vi "Streaming Message Loop.vi"(8 "error in (no error)":errorcluster, 9 "notifier out":refnum<notifier>, 10 "queue out":refnum<queue>, 11 "Message Queues":T1) -> (0 "error out":errorcluster)   [LabVIEW 2024]
doc: "The message loop subVI to handle messages pertaining to logging data."
uses:
  support/Message Queue/All Message Queues.ctl
  support/Message Queue/Message Cluster.ctl
  controls/DAQ_msgHandler StreamTypeDef.ctl
  CTRsample/Control/streamIO_states.ctl
  <vilib>/Utility/error.llb/Error Cluster From Error Code.vi
  <vilib>/ErrorRing/Error Ring.xnode
  support/Message Queue/DAQ_msgHandler Message Queue.lvlib
  Logging/DAQ_msgHandler Logging.lvlib
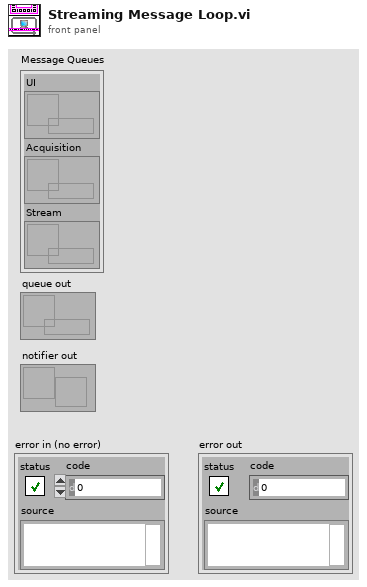
[diagram p1: front panel]
types:
  T1 = typedef "DAQ_msgHandler Message Queue.lvlib/All Message Queues.ctl" = cluster{"UI":refnum<queue>, "Acquisition":refnum<queue>, "Stream":refnum<queue>}
  T2 = typedef "streamIO_states.ctl" = enum16{"Fault", "Initialize", "Stream", "Close"}
  T3 = typedef "DAQ_msgHandler StreamTypeDef.ctl" = cluster{"stream state":T2, "CTR Node":string, "DAQ Node ID":i32, "Writer Endpoint":refnum<k21>, "Reader Endpoint":refnum<k21>, "Buffer":i32, "Managment Timeout":i32, "Stream Timeout":i32, "DAQ IP Addr":string, "CTR IP Addr":string, "Timeout Counter":i32}
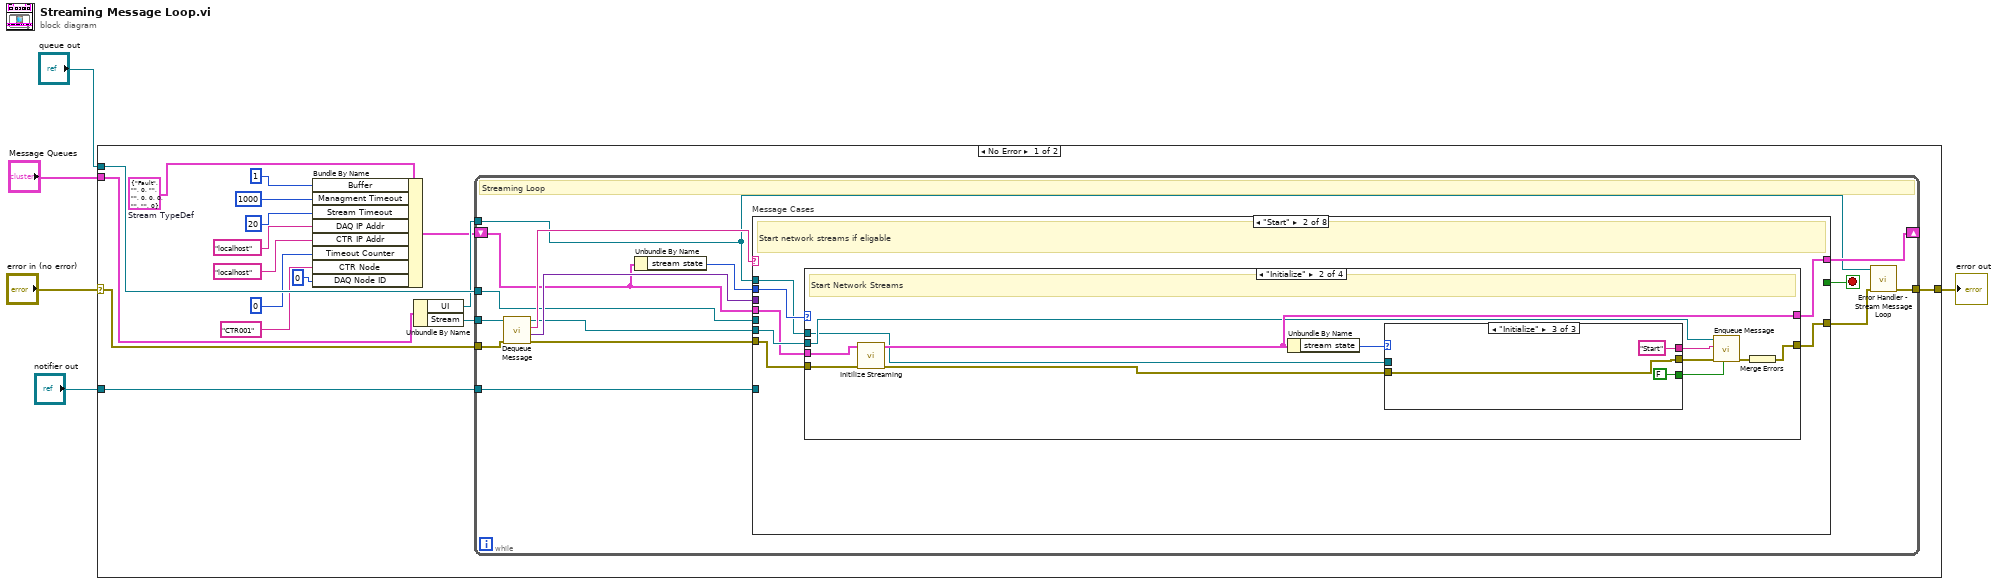
[diagram p0: block diagram]
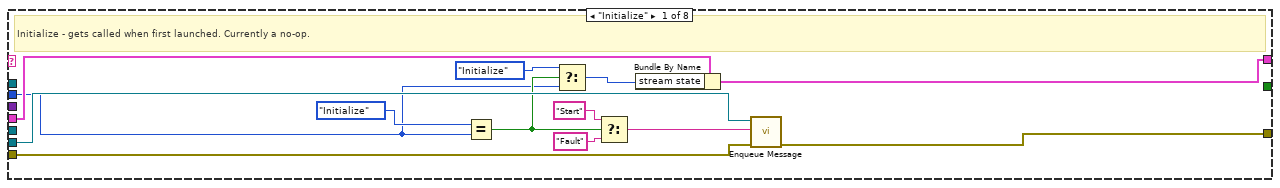
[diagram p2: hidden frame]
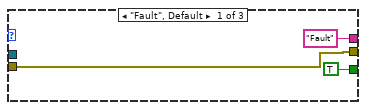
[diagram p4: hidden frame]
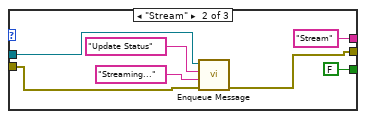
[diagram p5: hidden frame]
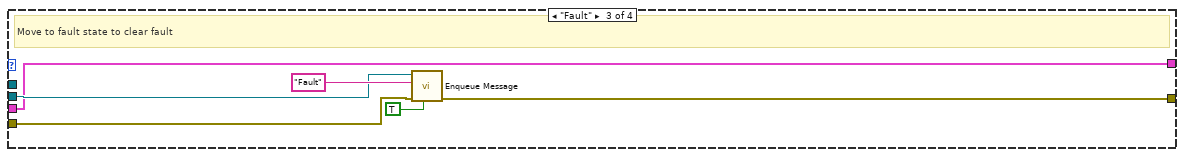
[diagram p6: hidden frame]
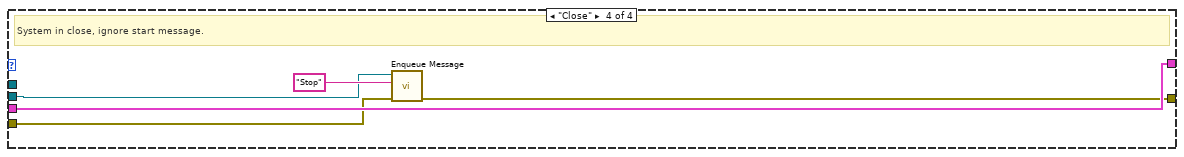
[diagram p7: hidden frame]
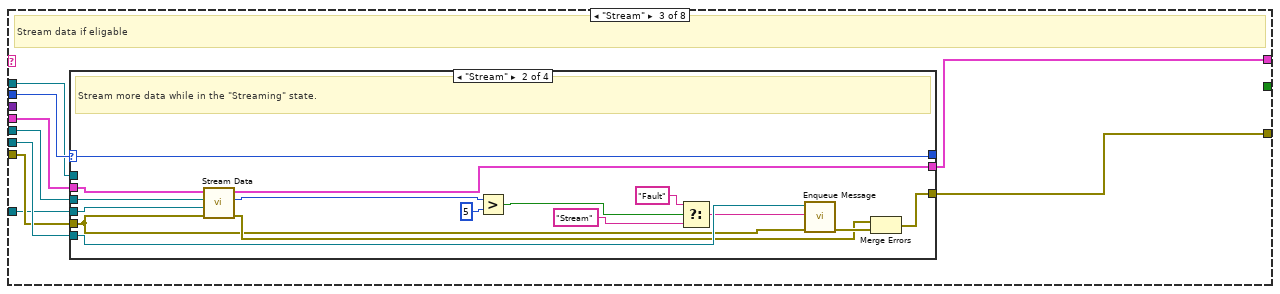
[diagram p8: hidden frame]
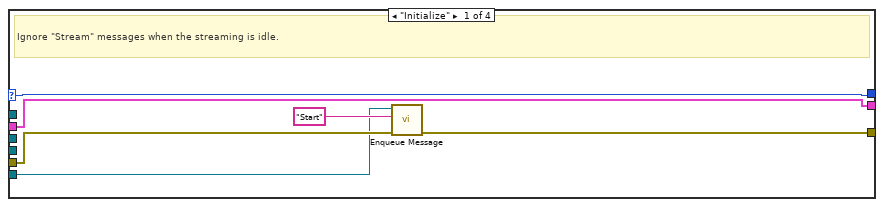
[diagram p9: hidden frame]
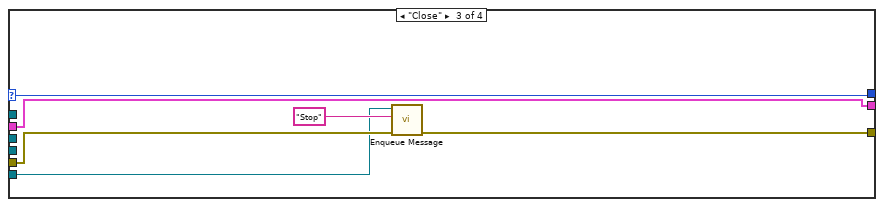
[diagram p10: hidden frame]
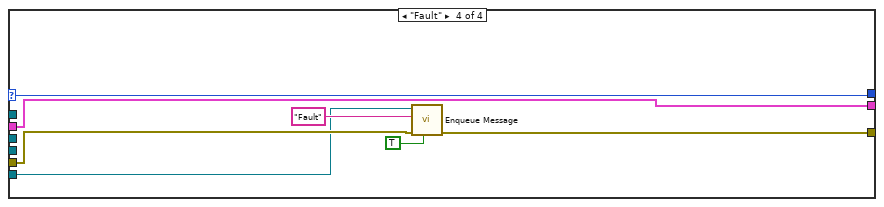
[diagram p11: hidden frame]
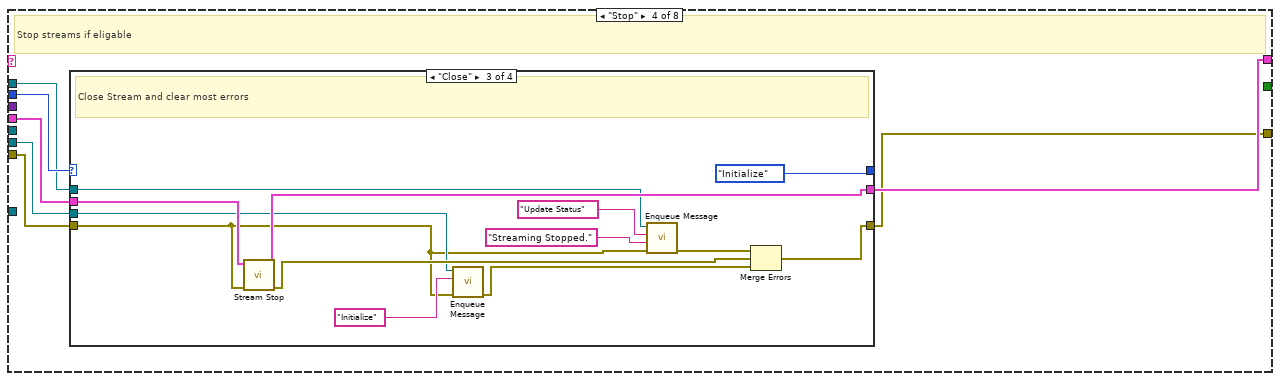
[diagram p12: hidden frame]
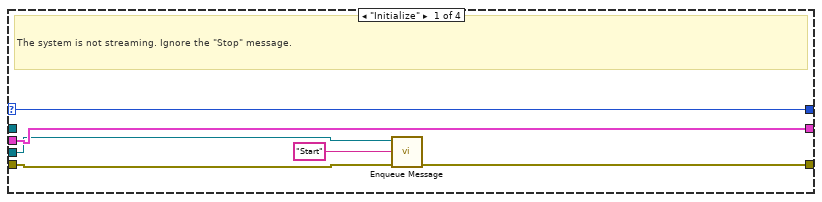
[diagram p13: hidden frame]
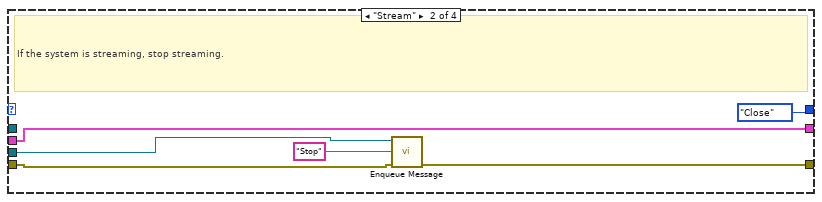
[diagram p14: hidden frame]
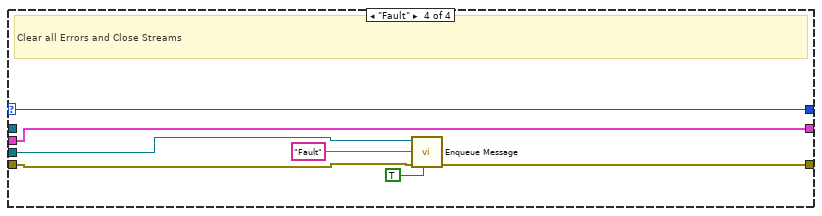
[diagram p15: hidden frame]
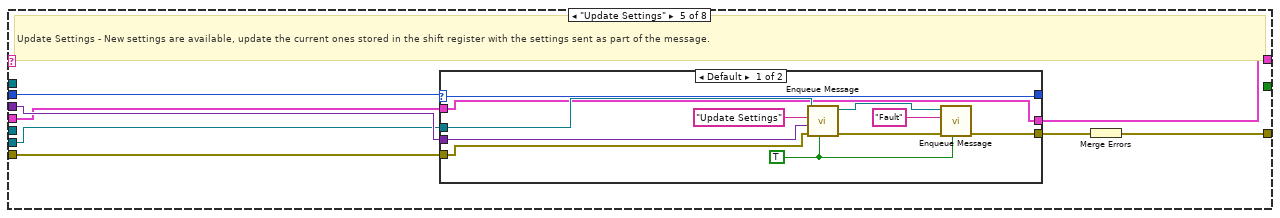
[diagram p16: hidden frame]
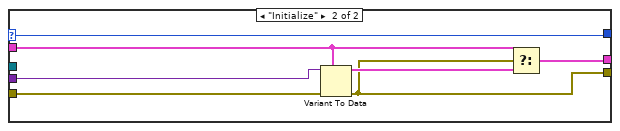
[diagram p17: hidden frame]
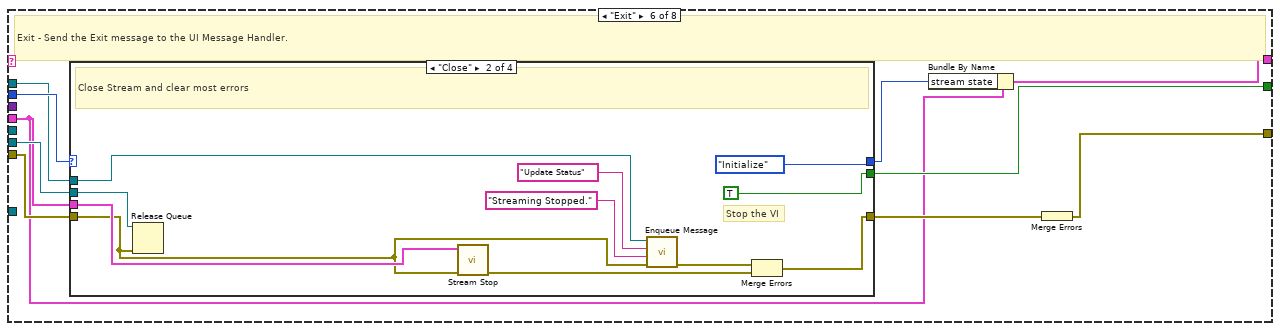
[diagram p18: hidden frame]
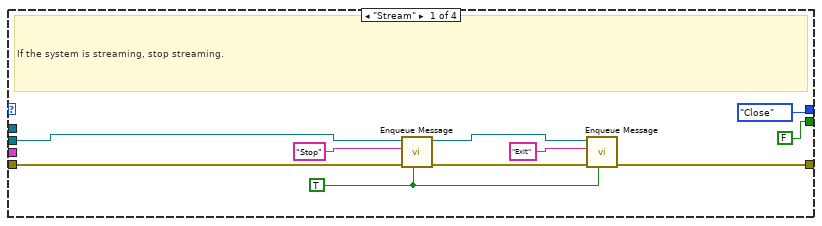
[diagram p19: hidden frame]
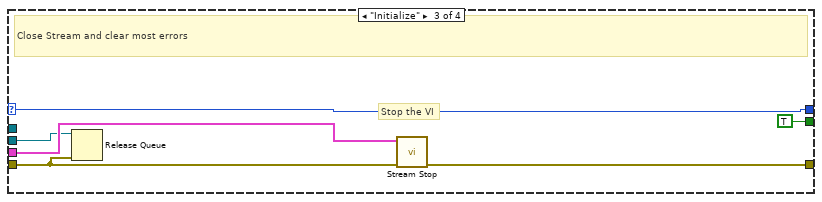
[diagram p20: hidden frame]
diagram:
  n1 = case shown="No Error" "error in (no error)" {
    selector: "error in (no error)" -> [w19 w286]
    tunnel: "Message Queues" -> [w22 _]
    tunnel: [w20 w286] -> w4
    tunnel: "queue out" -> [w18 _]
    tunnel: "notifier out" -> [w16 _]
    frame No Error {
      w15 = T3 {"stream state"=enum."Fault", "CTR Node"="", "DAQ Node ID"=0, "Writer Endpoint"="", "Reader Endpoint"="", "Buffer"=0, "Managment Timeout"=0, "Stream Timeout"=0, "DAQ IP Addr"="", "CTR IP Addr"="", "Timeout Counter"=0}  # Stream TypeDef
      n2 = Bundle By Name(cluster=w15, "Buffer"=1, "Managment Timeout"=1000, "Stream Timeout"=20, "DAQ IP Addr"="localhost", "CTR IP Addr"="localhost", "Timeout Counter"=0, "CTR Node"="CTR001", "DAQ Node ID"=0) -> (w14:T3)
      n3 = Unbundle By Name(w22) -> ("UI"=w17:refnum<queue>, "Stream"=w21:refnum<queue>)
      n4 = while {
        tunnel: w21 -> [w31]
        shift-right: [w25] -> _
        shift-left: w14 -> [w27]
        tunnel: w17 -> [w24]
        tunnel: w18 -> [w30]
        tunnel: w19 -> [w36]
        tunnel: [w29] -> w20
        tunnel: w16 -> [w28]
        stop <- w37 stop-if-true
        # "Streaming Loop"
        n5 = call "Dequeue Message.vi"("error in (no error)"=w36, "Message Queue"=w31) -> ("error out"=w35:errorcluster, "Message Data"=w33:variant, "Message"=w34:string, "dup Message Queue"=w32:refnum<queue>)  [unwired: 6 in]
        n6 = Unbundle By Name(w27) -> ("stream state"=w26:T2)
        n7 = case "Message Cases" shown="\"Start\"" w34 {
          selector: w34 -> [_ _ _ _ _ _ _ w277]
          tunnel: w32 -> [w48 w56 w103 w143 w180 w211 w262 w272]
          tunnel: w35 -> [w50 w55 w101 w145 w182 w212 w267 w276]
          tunnel: [w49 w57 w104 w141 w186 w214 w270 w275] -> w23
          tunnel: w27 -> [w47 w54 w100 w146 w184 w208 w268 w278]
          tunnel: [w46 w53 w97 w142 w183 w207 w265 w278] -> w25
          tunnel: [_ _ _ _ _ w210 _ _] -> w37
          tunnel: w33 -> [_ _ _ _ w185 _ _ _]
          tunnel: w30 -> [_ _ w102 _ _ _ _ _]
          tunnel: w26 -> [w39 w52 w99 w144 w181 w213 _ _]
          tunnel: w28 -> [_ _ w98 _ _ _ _ _]
          tunnel: w24 -> [_ w51 w96 w140 _ w205 w255 _]
          frame "Initialize" {
            # "Initialize - gets called when first launched. Currently a no-op."
            n8 = Equal?(x=streamIO_states."Initialize", y=w39) -> (x = y?=w40:bool)
            n9 = Select(t=streamIO_states."Initialize" ("stream state"), s=w40, f=w39) -> (s? t:f=w38:T2)
            n10 = Select(t="Start" ("Message"), s=w40, f="Fault") -> (s? t:f=w42:string)
            n11 = Bundle By Name(cluster=w47, "stream state"=w38) -> (w46:T3)
            n12 = call-poly "Enqueue Message.vi"("error in (no error)"=w50, "Message"=w42, "Message Queue"=w48) -> ("error out"=w49:errorcluster)  [unwired: 7 in, 1 out]
          }
          frame "Start" {
            # "Start network streams if eligable"
            n13 = case shown="\"Initialize\"" w52 {
              tunnel: [w58 w69 w87 w91] -> w57
              tunnel: w56 -> [_ w64 w89 w92]
              tunnel: w55 -> [w58 w68 w88 w93]
              tunnel: w54 -> [w59 w67 w85 w95]
              tunnel: [w59 w66 w85 w95] -> w53
              tunnel: w51 -> [_ w60 _ _]
              frame "Stream" {
                # "The system is already Streaming. Ignore the \"Start\" message."
              }
              frame "Initialize" {
                # "Start Network Streams"
                n14 = call "Initilize Streaming.vi"("error in (no error)"=w68, "DAQ_msgHandler StreamTypeDef"=w67) -> ("error out"=w62:errorcluster, "DAQ_msgHandler StreamTypeDef 2"=w66:T3)  [unwired: 8 in]
                n15 = Unbundle By Name(w66) -> ("stream state"=w65:T2)
                n16 = case shown="\"Initialize\"" w65 {
                  tunnel: ["Fault" ("Message") "Stream" ("Message") "Start" ("Message")] -> w71
                  tunnel: [TRUE ("Priority Message? (F)") FALSE ("Priority Message? (F)") FALSE ("Priority Message? (F)")] -> w63
                  tunnel: w62 -> [w72 w77 w82]
                  tunnel: [w72 w76 w82] -> w61
                  tunnel: w60 -> [_ w75 _]
                  frame "Fault", Default {
                  }
                  frame "Stream" {
                    n17 = call-poly "Enqueue Message.vi"("error in (no error)"=w77, "Message Data"="Streaming..." ("Acquiring and Logging..."), "Message"="Update Status", "Message Queue"=w75) -> ("error out"=w76:errorcluster)  [unwired: 6 in, 1 out]
                  }
                  frame "Initialize" {
                  }
                }
                n18 = call-poly "Enqueue Message.vi"("Priority Message? (F)"=w63, "error in (no error)"=w61, "Message"=w71, "Message Queue"=w64) -> ("error out"=w70:errorcluster)  [unwired: 6 in, 1 out]
                n19 = Merge Errors(w70) -> (w69:errorcluster)
              }
              frame "Fault" {
                # "Move to fault state to clear fault"
                n20 = call-poly "Enqueue Message.vi"("Priority Message? (F)"=TRUE, "error in (no error)"=w88, "Message"="Fault", "Message Queue"=w89) -> ("error out"=w87:errorcluster)  [unwired: 6 in, 1 out]
              }
              frame "Close" {
                # "System in close, ignore start message."
                n21 = call-poly "Enqueue Message.vi"("error in (no error)"=w93, "Message"="Stop", "Message Queue"=w92) -> ("error out"=w91:errorcluster)  [unwired: 7 in, 1 out]
              }
            }
          }
          frame "Stream" {
            # "Stream data if eligable"
            n22 = case shown="\"Stream\"" w99 {
              selector: w99 -> [w110 w121 w131 w138]
              tunnel: [w105 w126 w127 w133] -> w104
              tunnel: w103 -> [w106 w124 w128 w134]
              tunnel: w102 -> [_ w123 _ _]
              tunnel: w101 -> [w107 w111 w129 w135]
              tunnel: w100 -> [w109 w120 w132 w139]
              tunnel: [w110 w121 w131 w138] -> _
              tunnel: w98 -> [_ w119 _ _]
              tunnel: [w109 w118 w132 w139] -> w97
              tunnel: w96 -> [_ _ _ _]
              frame "Initialize" {
                # "Ignore \"Stream\" messages when the streaming is idle."
                n23 = call-poly "Enqueue Message.vi"("error in (no error)"=w107, "Message"="Start", "Message Queue"=w106) -> ("error out"=w105:errorcluster)  [unwired: 7 in, 1 out]
              }
              frame "Stream" {
                # "Stream more data while in the \"Streaming\" state."
                n24 = call "Stream Data.vi"("error in (no error)"=w111, "notifier out"=w119, "queue out"=w123, "DAQ_msgHandler StreamTypeDef"=w120) -> ("error out"=w122:errorcluster, "Timout Counter"=w112:i32, "DAQ_msgHandler StreamTypeDef 2"=w118:T3)  [unwired: 5 in]
                n25 = Greater?(x=w112, y=5 ("x")) -> (0:w116:bool)
                n26 = Select(t="Fault", s=w116, f="Stream" ("Message")) -> (s? t:f=w114:string)
                n27 = call-poly "Enqueue Message.vi"("error in (no error)"=w111, "Message"=w114, "Message Queue"=w124) -> ("error out"=w125:errorcluster)  [unwired: 7 in, 1 out]
                n28 = Merge Errors(w122, w125) -> (w126:errorcluster)
              }
              frame "Close" {
                n29 = call-poly "Enqueue Message.vi"("error in (no error)"=w129, "Message"="Stop", "Message Queue"=w128) -> ("error out"=w127:errorcluster)  [unwired: 7 in, 1 out]
              }
              frame "Fault" {
                n30 = call-poly "Enqueue Message.vi"("Priority Message? (F)"=TRUE, "error in (no error)"=w135, "Message"="Fault", "Message Queue"=w134) -> ("error out"=w133:errorcluster)  [unwired: 6 in, 1 out]
              }
            }
          }
          frame "Stop" {
            # "Stop streams if eligable"
            n31 = case shown="\"Close\"" w144 {
              selector: w144 -> [w152 _ _ w174]
              tunnel: [w148 w155 w168 w173] -> w141
              tunnel: w146 -> [w151 w153 w170 w172]
              tunnel: w145 -> [w149 w156 w161 w176]
              tunnel: [w152 streamIO_states."Close" ("stream state") streamIO_states."Initialize" ("stream state") w174] -> _
              tunnel: w143 -> [w147 w154 w165 w175]
              tunnel: [w151 w153 w169 w172] -> w142
              tunnel: w140 -> [_ _ w160 _]
              frame "Initialize" {
                # "The system is not streaming. Ignore the \"Stop\" message."
                n32 = call-poly "Enqueue Message.vi"("error in (no error)"=w149, "Message"="Start", "Message Queue"=w147) -> ("error out"=w148:errorcluster)  [unwired: 7 in, 1 out]
              }
              frame "Stream" {
                # "If the system is streaming, stop streaming."
                n33 = call-poly "Enqueue Message.vi"("error in (no error)"=w156, "Message"="Stop", "Message Queue"=w154) -> ("error out"=w155:errorcluster)  [unwired: 7 in, 1 out]
              }
              frame "Close" {
                # "Close Stream and clear most errors"
                n34 = call "Stream Stop.vi"("error in (no error)"=w161, "DAQ_msgHandler StreamTypeDef"=w170) -> ("error out"=w167:errorcluster, "DAQ_msgHandler StreamTypeDef 2"=w169:T3)  [unwired: 8 in]
                n35 = call-poly "Enqueue Message.vi"("error in (no error)"=w161, "Message"="Initialize", "Message Queue"=w165) -> ("error out"=w164:errorcluster)  [unwired: 7 in, 1 out]
                n36 = call-poly "Enqueue Message.vi"("error in (no error)"=w161, "Message Data"="Streaming Stopped." ("Acquiring and Logging..."), "Message"="Update Status", "Message Queue"=w160) -> ("error out"=w159:errorcluster)  [unwired: 6 in, 1 out]
                n37 = Merge Errors(w159, w167, w164) -> (w168:errorcluster)
              }
              frame "Fault" {
                # "Clear all Errors and Close Streams"
                n38 = call-poly "Enqueue Message.vi"("Priority Message? (F)"=TRUE, "error in (no error)"=w176, "Message"="Fault", "Message Queue"=w175) -> ("error out"=w173:errorcluster)  [unwired: 6 in, 1 out]
              }
            }
          }
          frame "Update Settings" {
            # "Update Settings - New settings are available, update the current ones stored in the shift register with the settings sent as part of the message."
            n39 = case shown="Default" w181 {
              selector: w181 -> [w187 w198]
              tunnel: w185 -> [w188 w204]
              tunnel: w184 -> [w190 w203]
              tunnel: [w190 w201] -> w183
              tunnel: w182 -> [w195 w200]
              tunnel: w180 -> [w196 _]
              tunnel: [w191 w199] -> w179
              tunnel: [w187 w198] -> _
              frame Default {
                w189 = TRUE ("Priority Message? (F)")
                n40 = call-poly "Enqueue Message.vi"("Priority Message? (F)"=w189, "error in (no error)"=w195, "Message Data"=w188, "Message"="Update Settings", "Message Queue"=w196) -> ("error out"=w194:errorcluster, "dup Message Queue"=w193:refnum<queue>)  [unwired: 5 in]
                n41 = call-poly "Enqueue Message.vi"("Priority Message? (F)"=w189, "error in (no error)"=w194, "Message"="Fault", "Message Queue"=w193) -> ("error out"=w191:errorcluster)  [unwired: 6 in, 1 out]
              }
              frame "Initialize" {
                n42 = Variant To Data(error in=w200, type=w203, Variant=w204) -> (data=w202:T3, error out=w199:errorcluster)
                n43 = Select(t=w203, s=w199, f=w202) -> (s? t:f=w201:T3)
              }
            }
            n44 = Merge Errors(w179) -> (w186:errorcluster)
          }
          frame "Exit" {
            # "Exit - Send the Exit message to the UI Message Handler."
            n45 = case shown="\"Close\"" w213 {
              selector: w213 -> [_ _ w236 w242]
              tunnel: [w217 w225 w240 w244] -> w209
              tunnel: w208 -> [_ w235 w241 _]
              tunnel: w212 -> [w223 w229 w237 w250]
              tunnel: w211 -> [w222 w234 w239 w249]
              tunnel: [FALSE TRUE TRUE FALSE] -> w210
              tunnel: [streamIO_states."Close" ("stream state") streamIO_states."Initialize" ("stream state") w236 w242] -> w206
              tunnel: w205 -> [_ w228 _ _]
              frame "Stream" {
                w215 = TRUE ("Priority Message? (F)")
                # "If the system is streaming, stop streaming."
                n46 = call-poly "Enqueue Message.vi"("Priority Message? (F)"=w215, "error in (no error)"=w223, "Message"="Stop", "Message Queue"=w222) -> ("error out"=w220:errorcluster, "dup Message Queue"=w219:refnum<queue>)  [unwired: 6 in]
                n47 = call-poly "Enqueue Message.vi"("Priority Message? (F)"=w215, "error in (no error)"=w220, "Message"="Exit", "Message Queue"=w219) -> ("error out"=w217:errorcluster)  [unwired: 6 in, 1 out]
              }
              frame "Close" {
                # "Stop the VI"
                # "Close Stream and clear most errors"
                n48 = Release Queue(queue=w234, error in (no error)=w229) -> ()  [unwired: 1 in, 3 out]
                n49 = call "Stream Stop.vi"("error in (no error)"=w229, "DAQ_msgHandler StreamTypeDef"=w235) -> ("error out"=w227:errorcluster)  [unwired: 8 in, 1 out]
                n50 = call-poly "Enqueue Message.vi"("error in (no error)"=w229, "Message Data"="Streaming Stopped." ("Acquiring and Logging..."), "Message"="Update Status", "Message Queue"=w228) -> ("error out"=w226:errorcluster)  [unwired: 6 in, 1 out]
                n51 = Merge Errors(w226, w227) -> (w225:errorcluster)
              }
              frame "Initialize" {
                # "Stop the VI"
                # "Close Stream and clear most errors"
                n52 = Release Queue(queue=w239, error in (no error)=w237) -> ()  [unwired: 1 in, 3 out]
                n53 = call "Stream Stop.vi"("error in (no error)"=w237, "DAQ_msgHandler StreamTypeDef"=w241) -> ("error out"=w240:errorcluster)  [unwired: 8 in, 1 out]
              }
              frame "Fault" {
                w243 = TRUE ("Priority Message? (F)")
                # "Clear all Errors and Close Streams"
                n54 = call-poly "Enqueue Message.vi"("Priority Message? (F)"=w243, "error in (no error)"=w250, "Message"="Exit", "Message Queue"=w249) -> ("error out"=w247:errorcluster, "dup Message Queue"=w246:refnum<queue>)  [unwired: 6 in]
                n55 = call-poly "Enqueue Message.vi"("Priority Message? (F)"=w243, "error in (no error)"=w247, "Message"="Fault", "Message Queue"=w246) -> ("error out"=w244:errorcluster)  [unwired: 6 in, 1 out]
              }
            }
            n56 = Bundle By Name(cluster=w208, "stream state"=w206) -> (w207:T3)
            n57 = Merge Errors(w209) -> (w214:errorcluster)
          }
          frame "Fault" {
            # "Clear everything and start fresh"
            n58 = Flush Queue(queue=w262) -> (queue out=w261:refnum<queue>)  [unwired: 1 in, 2 out]
            n59 = call "Stream Stop.vi"("error in (no error)"=w267, "DAQ_msgHandler StreamTypeDef"=w268) -> ("error out"=w269:errorcluster, "DAQ_msgHandler StreamTypeDef 2"=w266:T3)  [unwired: 8 in]
            n60 = call <vilib>:"Clear Errors.vi"("error in (no error)"=w269) -> ("error out"=w264:errorcluster)  [unwired: 5 in, 1 out]
            n61 = Bundle By Name(cluster=w266, "stream state"=streamIO_states."Initialize") -> (w265:T3)
            n62 = call "Enqueue Message (Single).vi"("error in (no error)"=w264, "Message"="Initialize", "Message Queue"=w261) -> ("error out"=w259:errorcluster)  [unwired: 7 in, 1 out]
            n63 = call "Enqueue Message (Single).vi"("error in (no error)"=w259, "Message"="Broadcast settings", "Message Queue"=w255) -> ("error out"=w253:errorcluster, "dup Message Queue"=w254:refnum<queue>)  [unwired: 7 in]
            n64 = call-poly "Enqueue Message.vi"("error in (no error)"=w253, "Message Data"="Streaming Faulted." ("Acquiring and Logging..."), "Message"="Update Status", "Message Queue"=w254) -> ("error out"=w252:errorcluster)  [unwired: 6 in, 1 out]
            n65 = Merge Errors(w252) -> (w270:errorcluster)
          }
          frame Default {
            # "'Default' case only runs if there is a message that isn't defined in any of the other cases.  Output a programming error."
            n66 = xnode "Error Ring"("parameter 0"=w277) -> ("error out"=w274:errorcluster)
            n67 = call "Enqueue Message (Single).vi"("error in (no error)"=w276, "Message"="Fault", "Message Queue"=w272) -> ("error out"=w273:errorcluster)  [unwired: 7 in, 1 out]
            n68 = Merge Errors(w274, w273) -> (w275:errorcluster)
          }
        }
        n69 = call "Error Handler - Stream Message Loop.vi"("error in (no error)"=w23, "Message Queue"=w24) -> ("dup error in"=w29:errorcluster)  [unwired: 8 in, 1 out]
      }
    }
    frame Error {
    }
  }
  "error out" <- w4
